vi "Climb.vi"(11 "Start":bool) -> ()   [LabVIEW 2015]
panel:
  in  "Button":bool
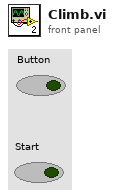
[diagram p1: front panel]
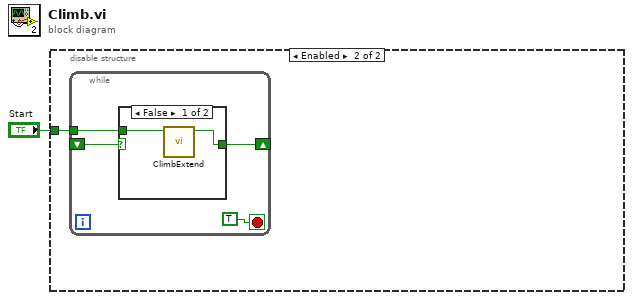
[diagram p0: block diagram]
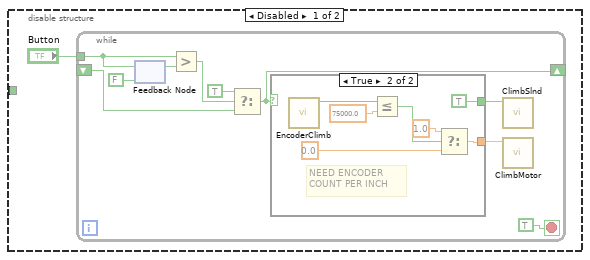
[diagram p2: hidden frame]
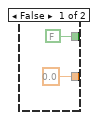
[diagram p3: hidden frame]
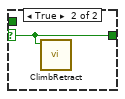
[diagram p4: hidden frame]
diagram:
  n1 = disable-structure shown="Enabled" {
    disable-tunnel: "Start" -> [_ w22]
    frame Disabled {
      n2 = while {
        tunnel: "Button" -> [w11]
        shift-right: [w9] -> _
        shift-left: _ -> [w10]
        stop <- TRUE stop-if-true
        n3 = feedback #1(FALSE) -> (w6:bool)
        n4 = feedback-in #1(w11) -> ()
        n5 = Greater?(x=w11, y=w6) -> (0:w5:bool)
        n6 = Select(t=TRUE, s=w5, f=w10) -> (s? t:f=w9:bool)
        n7 = case shown="True" w9 {
          tunnel: [FALSE TRUE] -> w8
          tunnel: [0.0 w15] -> w3
          frame False {
          }
          frame True {
            # "NEED ENCODER\nCOUNT PER INCH"
            n8 = call "EncoderClimb.vi"() -> ("Position_out"=w21:i32)  [unwired: 11 in]
            n9 = Less Or Equal?(x=w21, y=75000.0) -> (x <= y?=w18:bool)
            n10 = Select(t=1.0, s=w18, f=0.0) -> (s? t:f=w15:dbl)
          }
        }
        n11 = call "ClimbSlnd.vi"("Button"=w8) -> ()  [unwired: 11 in]
        n12 = call "ClimbMotor.vi"("Power"=w3) -> ()  [unwired: 11 in]
      }
    }
    frame Enabled {
      n13 = while {
        shift-right: [w24] -> _
        shift-left: _ -> [w25]
        tunnel: w22 -> [w23]
        stop <- TRUE stop-if-true
        n14 = case shown="False" w25 {
          selector: w25 -> [_ w29]
          tunnel: [w28 w29] -> w24
          tunnel: w23 -> [w27 _]
          frame False {
            n15 = call "ClimbExtend.vi"("Button"=w27) -> ("Complete?"=w28:bool)  [unwired: 10 in]
          }
          frame True {
            n16 = call "ClimbRetract.vi"("Button"=w29) -> ()  [unwired: 10 in, 1 out]
          }
        }
      }
    }
  }
